vi "strToArrayValue.vi"(8 "error in (no error)":errorcluster, 10 "String":string, 11 "MatOper in":refnum<class "MatOper.lvclass">) -> (0 "error out":errorcluster, 2 "Array":dbl[](array[numeric]), 3 "MatOper out":refnum<class "MatOper.lvclass">)   [LabVIEW 2016, in "OfcFunc.lvlib" / "MatOper.lvclass"]
doc: "Get the string data as the array."
uses:
  MatOper.lvclass
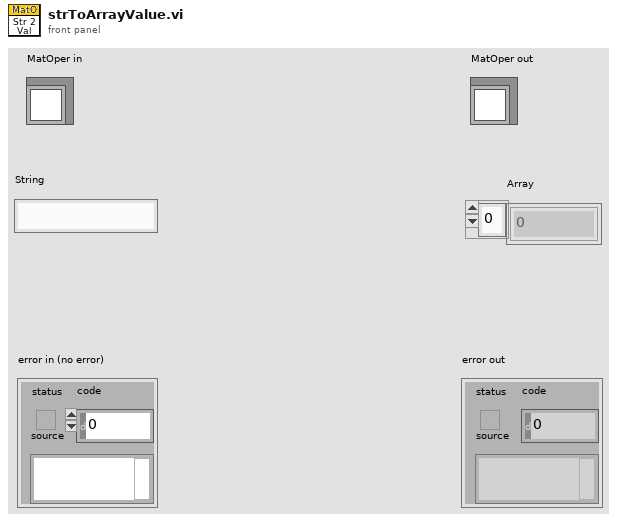
[diagram p1: front panel]
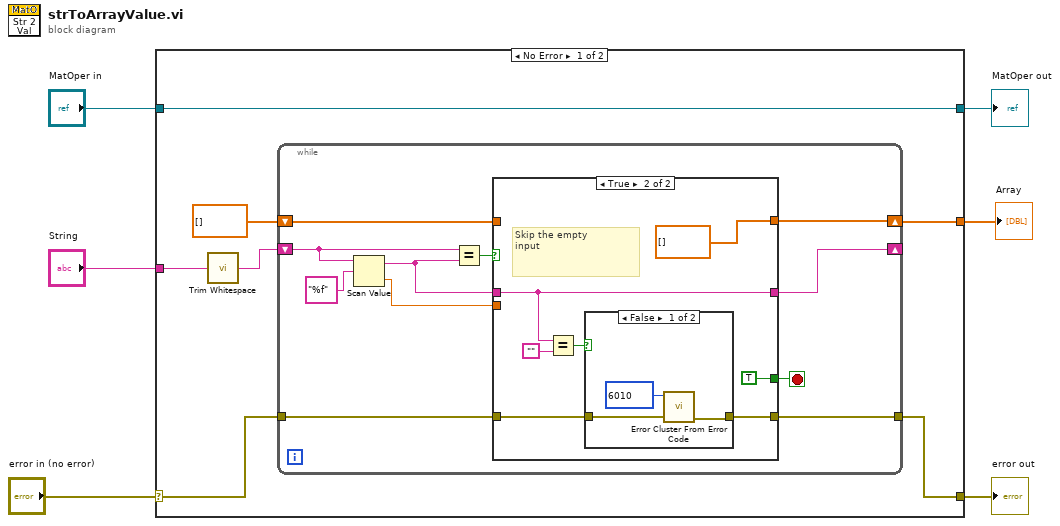
[diagram p0: block diagram]
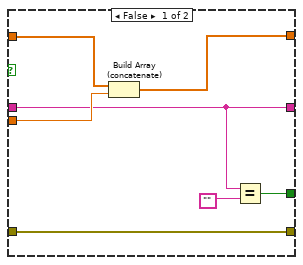
[diagram p2: hidden frame]
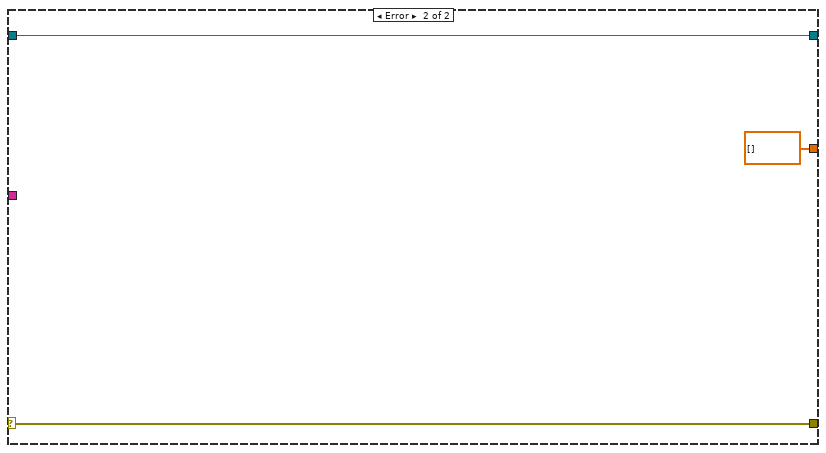
[diagram p4: hidden frame]
diagram:
  n1 = case shown="No Error" "error in (no error)" {
    selector: "error in (no error)" -> [w9 w45]
    tunnel: [w10 w45] -> w5
    tunnel: [w13 w44] -> w3
    tunnel: "MatOper in" -> [w13 w44]
    tunnel: [w8 dbl[] []] -> w2
    tunnel: "String" -> [w7 _]
    frame No Error {
      n2 = call <vilib>:"Trim Whitespace.vi"("string"=w7) -> ("trimmed string"=w11:string)  [unwired: 1 in]
      n3 = while {
        shift-right: [w20] -> _
        shift-left: w11 -> [w15]
        shift-right: [w22] -> w8
        shift-left: dbl[] [] -> [w23]
        tunnel: [w18] -> w10
        tunnel: w9 -> [w17]
        stop <- w19 stop-if-true
        n4 = Scan Value(string=w15, format string="%f") -> (output string=w16:string, value=w21:dbl)  [unwired: 1 in]
        n5 = Equal?(x=w15, y=w16) -> (x = y?=w14:bool)
        n6 = case shown="True" w14 {
          tunnel: [w29 dbl[] []] -> w22
          tunnel: w23 -> [w30 _]
          tunnel: w21 -> [w31 _]
          tunnel: w16 -> [w27 w35]
          tunnel: [w27 w35] -> w20
          tunnel: [w26 TRUE] -> w19
          tunnel: [w25 w32] -> w18
          tunnel: w17 -> [w25 w33]
          frame False {
            n7 = Build Array (concatenate)(w30, w31) -> (w29:dbl[])
            n8 = Equal?(x=w27, y="") -> (x = y?=w26:bool)
          }
          frame True {
            # "Skip the empty\ninput"
            n9 = Equal?(x=w35, y="") -> (x = y?=w36:bool)
            n10 = case shown="False" w36 {
              tunnel: w33 -> [w40 w42]
              tunnel: [w39 w42] -> w32
              frame False {
                n11 = call <vilib>:"Error Cluster From Error Code.vi"("error in (no error)"=w40, "error code (0)"=6010) -> ("error out"=w39:errorcluster)  [unwired: 7 in]
              }
              frame True {
              }
            }
          }
        }
      }
    }
    frame Error {
    }
  }
  "error out" <- w5
  "MatOper out" <- w3
  "Array" <- w2
